vi "test_ParseSolutionFile_EmptyFile.vi"() -> (3 "Pass?":bool)   [LabVIEW 2019, in "Tests.SolutionBuilder.lvlib"]
uses:
  Tests.SolutionBuilder.lvlib
  SolutionBuilder/SolutionBuilder.lvclass
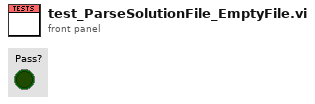
[diagram p1: front panel]
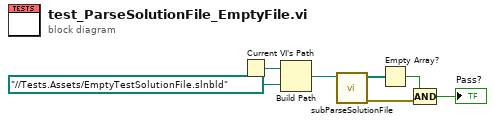
[diagram p0: block diagram]
diagram:
  n1 = Current VI's Path() -> (path=w4:path)
  n2 = Build Path(base path=w4, name or relative path=path "../../Tests.Assets/EmptyTestSolutionFile.slnbld" ("Path")) -> (appended path=w3:path)
  n3 = call "subParseSolutionFile.vi"("Solution file"=w3) -> ("error out"=w1:errorcluster, "Projects"=w2:path[])  [unwired: 7 in, 2 out]
  n4 = Empty Array?(array=w2) -> (empty?=w6:bool)
  n5 = Compound Arithmetic op=AND(w6, w1) -> (→"Pass?":bool)
